vi "array_reverse_whileloop.vi"() -> ()   [LabVIEW 2020]
panel:
  out "Reverse":dbl[](array[numeric])
  out "Original":dbl[](array[numeric])
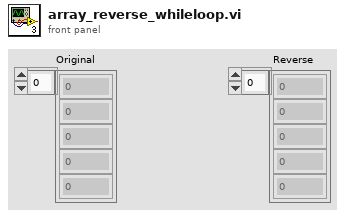
[diagram p1: front panel]
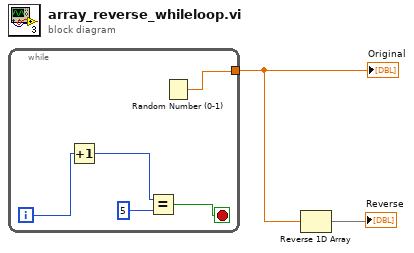
[diagram p0: block diagram]
diagram:
  n1 = while {
    tunnel: [w3] -> w2
    i -> [w6]
    stop <- w4 stop-if-true
    n2 = Increment(x=w6) -> (x+1=w5:i32)
    n3 = Equal?(x=w5, y=5) -> (x = y?=w4:bool)
    n4 = Random Number (0-1)() -> (number: 0 to 1=w3:dbl)
  }
  "Original" <- w2
  n5 = Reverse 1D Array(array=w2) -> (reversed array=→"Reverse":dbl[])
